vi "SRV_PM_Add Packet Data.vi"(9 "New Packet Data":u8[](array[numeric]) format="%.0x", 10 "Packet Data":u8[](array[numeric]) format="%.0x") -> (2 "Packet Data out":u8[](array[numeric]) format="%.0x")   [LabVIEW 2014]
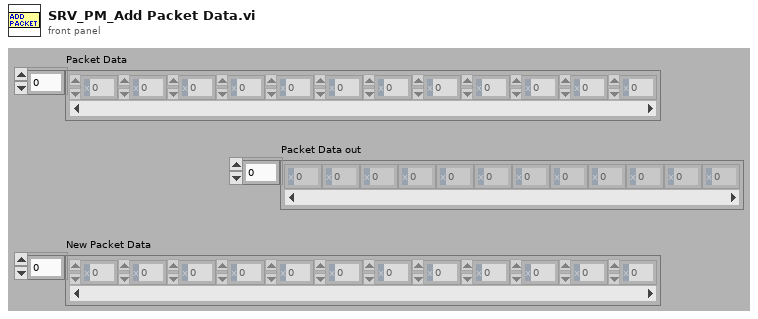
[diagram p1: front panel]
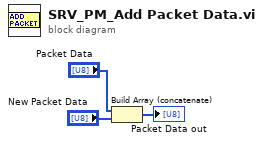
[diagram p0: block diagram]
diagram:
  n1 = Build Array (concatenate)("Packet Data", "New Packet Data") -> (→"Packet Data out":u8[])
